vi "Main UI.vi"(11 "FormulaLV App in":refnum<class "FormulaG App.lvclass">) -> ()   [LabVIEW 2020, in "FormulaG.lvlib" / "FormulaG App.lvclass"]
uses:
  FormulaG App.lvclass
  FormulaG-Common/Camera.ctl
  <vilib>/sklein/WebView2/Webview2 Control/WebView2 Control.xctl
  FormulaG App.lvclass/FormulaG App.ctl
  FormulaG-Common/UI Options.ctl
  <vilib>/Platform/browser.llb/Open URL in Default Browser (string).vi
  HTTP Logs UI.vi
  FormulaG-Common/FormulaG-Common.lvlib
  FormulaG API/FormulaG API.lvclass
  <vilib>/IlluminatedG/IG GodotServer/GodotLV/GodotServer/GodotServer.lvclass
panel:
  out "Web":string(xcontrol)
  in  "HTTP Logs":bool
  out "Throttle":sgl(slide) scale=0.0..1.0
  out "Speed":dbl(knob) scale=0.0..10.0
  in  "Clear Map":bool
  out "Last Lap":dbl format="%<%M:%S%3u>t"
  out "Current Lap":dbl format="%<%M:%S%3u>t"
  out "XY Graph":cluster{dbl[], dbl[]}[](graph)
  in  "Pause":bool
  out "Chart":sgl[][](graph)
  in  "Camera":T1
  in  "Reset":bool
  out "Steering":sgl(knob) scale=-1.0..1.0
  out "Connected":bool
  in  "Show Range Lines":bool
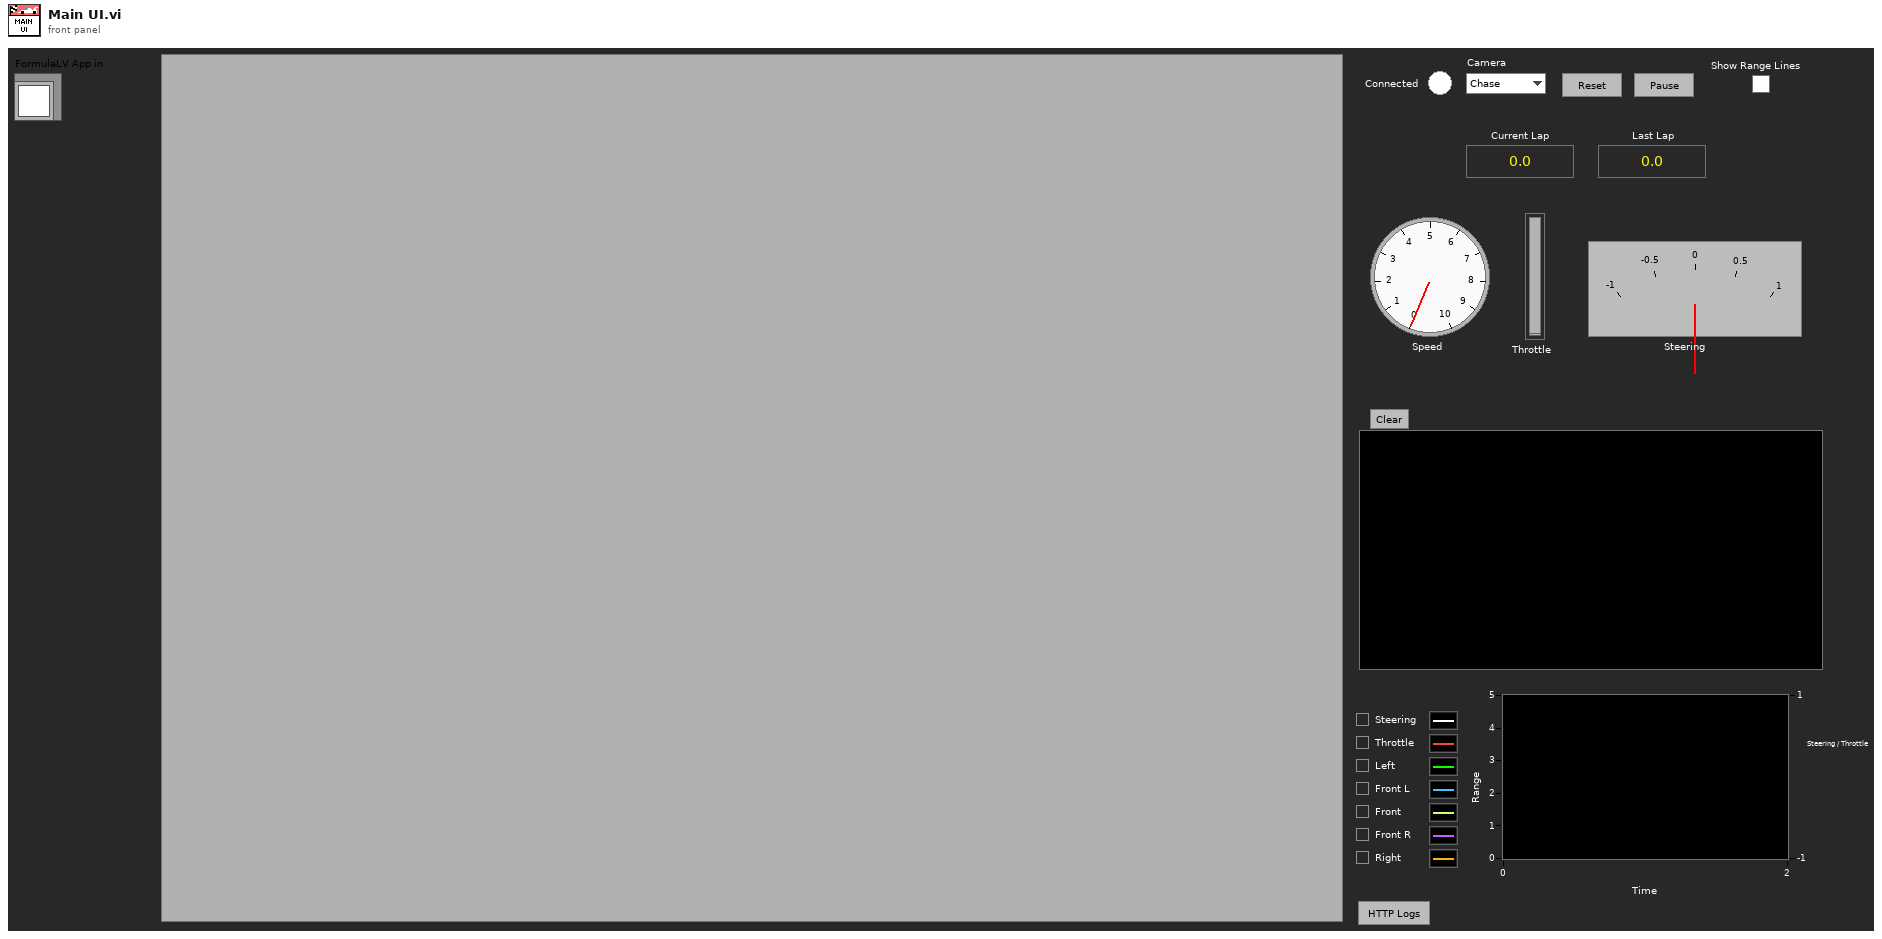
[diagram p1: front panel]
types:
  T1 = typedef "FormulaG-Common.lvlib/Camera.ctl" = enum16{"Chase", "Overhead"}
  T2 = typedef "FormulaG-Common.lvlib/UI Options.ctl" = cluster{"Range Visible":bool}
  T3 = typedef "FormulaG-Common.lvlib/Control VI.ctl" = refnum<vi>
  T4 = typedef "FormulaG-Common.lvlib/Ranges.ctl" = cluster{"Front":sgl[], "Rear":sgl[]}
  T5 = typedef "FormulaG-Common.lvlib/Car Info.ctl" = cluster{"Speed":sgl, "X":sgl, "Y":sgl, "Heading":sgl}
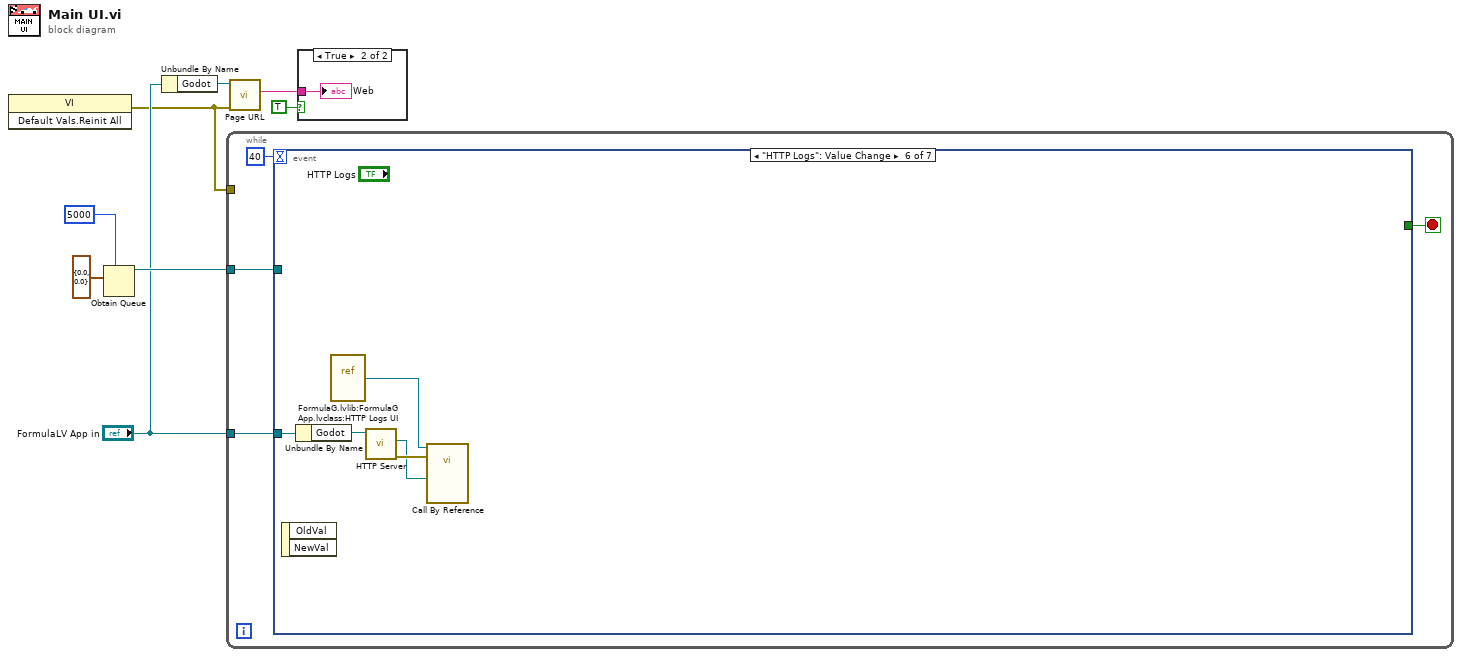
[diagram p0: block diagram]
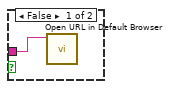
[diagram p2: hidden frame]
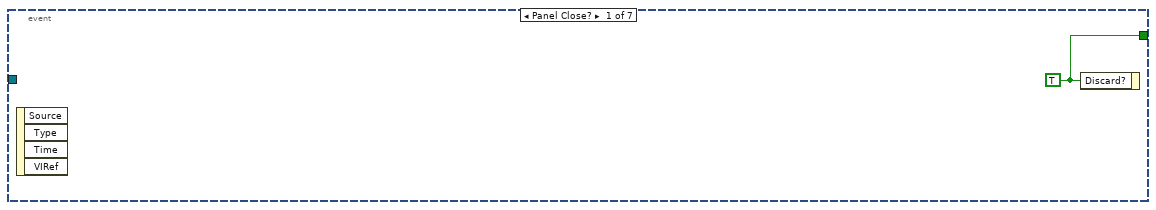
[diagram p3: hidden frame]
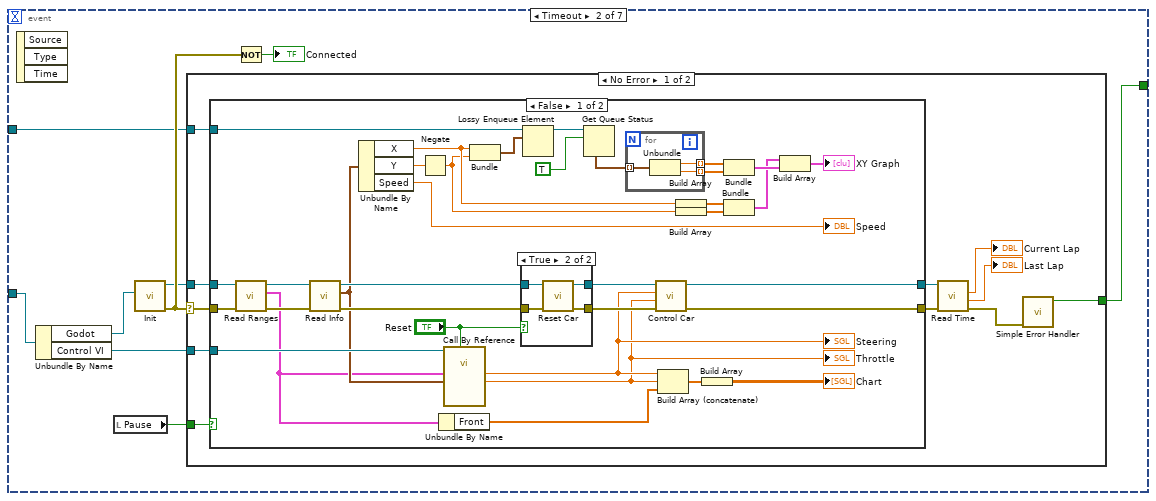
[diagram p4: hidden frame]
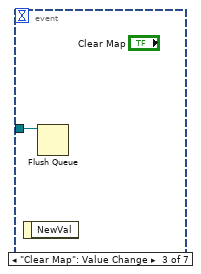
[diagram p8: hidden frame]
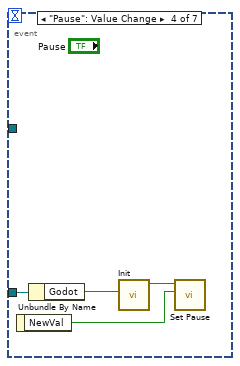
[diagram p9: hidden frame]
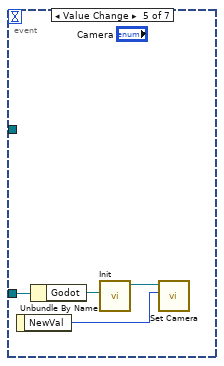
[diagram p10: hidden frame]
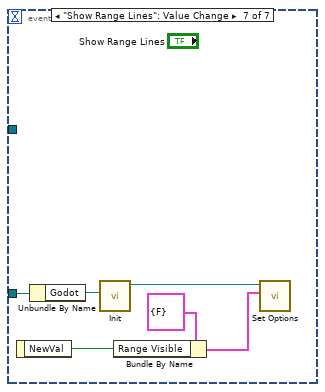
[diagram p11: hidden frame]
diagram:
  n1 = invoke class="VI" method="Default Vals.Reinit All"() -> (error out=w1:errorcluster)  [unwired: 3 in, 2 out]
  n2 = Obtain Queue(max queue size (-1, unlimited)=5000, element data type=cluster{dbl, dbl} {0.0, 0.0}) -> (queue out=w6:refnum<queue>)  [unwired: 3 in, 2 out]
  n3 = Unbundle By Name("FormulaLV App in") -> ("Godot"=w3:refnum<class "GodotServer.lvclass">)
  n4 = while {
    tunnel: "FormulaLV App in" -> [w11]
    tunnel: w1 -> [_]
    tunnel: w6 -> [w9]
    stop <- w12 stop-if-true
    n5 = event shown="[5] \"HTTP Logs\": Value Change" {
      selector: _ -> [_ _ _ _ _ _ _]
      dyn-events: _ -> [_ _ _ _ _ _ _]
      timeout: 40 -> [_ _ _ _ _ _ _]
      tunnel: [w13 w16 _ _ _ _ _] -> w12
      tunnel: w11 -> [_ w18 _ w83 w87 w92 w98]
      tunnel: w9 -> [_ w19 w79 _ _ _ _]
      event Panel Close? {
        w13 = TRUE ("Discard?")
        n6 = event-data() -> ()  [unwired: 1 in, 4 out]
        n7 = event-data("Discard?"=w13) -> ()  [unwired: 1 in, 1 out]
      }
      event Timeout {
        n8 = event-data() -> ()  [unwired: 1 in, 3 out]
        n9 = Unbundle By Name(w18) -> ("Godot"=w14:refnum<class "GodotServer.lvclass">, "Control VI"=w17:T3)
        n10 = local read "Pause"() -> (w15:bool)
        n11 = call "Init.vi"("Godot"=w14) -> ("error out"=w21:errorcluster, "FormulaG API out"=w20:refnum<class "FormulaG API.lvclass">)  [unwired: 9 in]
        n12 = case shown="No Error" w21 {
          selector: w21 -> [w30 _]
          tunnel: w20 -> [w33 _]
          tunnel: w19 -> [w32 _]
          tunnel: w17 -> [w31 _]
          tunnel: [w28 _] -> w16
          tunnel: w15 -> [w29 _]
          frame No Error {
            n13 = case shown="False" w29 {
              tunnel: w33 -> [w65 w78]
              tunnel: w32 -> [w61 _]
              tunnel: w31 -> [w47 _]
              tunnel: w30 -> [w39 _]
              tunnel: [w35 w78] -> w27
              tunnel: [w34 _] -> w26
              frame False {
                n14 = call "Read Ranges.vi"("error in (no error)"=w39, "FormulaG API in"=w65) -> ("error out"=w66:errorcluster, "Ranges"=w45:T4, "FormulaG API out"=w64:refnum<class "FormulaG API.lvclass">)  [unwired: 7 in]
                n15 = call "Read Info.vi"("error in (no error)"=w66, "FormulaG API in"=w64) -> ("error out"=w68:errorcluster, "Info"=w46:T5, "FormulaG API out"=w63:refnum<class "FormulaG API.lvclass">)  [unwired: 7 in]
                n16 = Unbundle By Name(w46) -> ("X"=w57:sgl, "Y"=w62:sgl, "Speed"=→"Speed":sgl)
                n17 = Negate(x=w62) -> (-x=w56:sgl)
                n18 = Unbundle By Name(w45) -> ("Front"=w44:sgl[])
                n19 = call-by-ref "?"(reference=w47, "Reset"="Reset", "Car Info"=w46, "Ranges"=w45) -> ("Throttle (0 to 1)"=w37:sgl, "Steering (-1 to 1)"=w41:sgl)  [unwired: 8 in, 2 out]
                "Steering" <- w41
                "Throttle" <- w37
                n20 = Bundle("X"=w57, w56) -> (w60:cluster{"X":sgl, sgl})  [unwired: 1 in]
                n21 = case shown="True" "Reset" {
                  tunnel: w63 -> [w70 w74]
                  tunnel: [w70 w73] -> w40
                  tunnel: w68 -> [w69 w72]
                  tunnel: [w69 w71] -> w67
                  frame False {
                  }
                  frame True {
                    n22 = call "Reset Car.vi"("error in (no error)"=w72, "FormulaG API in"=w74) -> ("error out"=w71:errorcluster, "FormulaG API out"=w73:refnum<class "FormulaG API.lvclass">)  [unwired: 8 in]
                  }
                }
                n23 = Lossy Enqueue Element(queue=w61, element=w60) -> (queue out=w59:refnum<queue>)  [unwired: 1 in, 3 out]
                n24 = Get Queue Status(queue=w59, return elements? (F)=TRUE) -> (elements=w55:cluster{dbl, dbl}[])  [unwired: 1 in, 7 out]
                n25 = for {
                  tunnel: w55 -> [w77] mode=indexing
                  tunnel: [w76] -> w52 mode=indexing
                  tunnel: [w75] -> w51 mode=indexing
                  n26 = Unbundle(w77) -> (w76:dbl, w75:dbl)
                }
                n27 = call "Control Car.vi"("error in (no error)"=w67, "Throttle"=w37, "Steering"=w41, "FormulaG API in"=w40) -> ("error out"=w34:errorcluster, "FormulaG API out"=w35:refnum<class "FormulaG API.lvclass">)  [unwired: 6 in]
                n28 = Build Array (concatenate)(w41, w37, w44) -> (w43:sgl[])
                n29 = Build Array(w57) -> (w54:sgl[])
                n30 = Build Array(w56) -> (w53:sgl[])
                n31 = Build Array(w43) -> (→"Chart":sgl[][])
                n32 = Bundle(w52, w51) -> (w50:cluster{dbl[], dbl[]})  [unwired: 1 in]
                n33 = Bundle(w54, w53) -> (w49:cluster{sgl[], sgl[]})  [unwired: 1 in]
                n34 = Build Array(w49, w50) -> (→"XY Graph":cluster{dbl[], dbl[]}[])
              }
              frame True {
              }
            }
            n35 = call "Read Time.vi"("error in (no error)"=w26, "FormulaG API in"=w27) -> ("error out"=w25:errorcluster, "Last Lap"=→"Last Lap":dbl, "Current Lap"=→"Current Lap":dbl)  [unwired: 6 in, 1 out]
            n36 = call <vilib>:"Simple Error Handler.vi"("error in (no error)"=w25) -> ("error?"=w28:bool)  [unwired: 4 in, 4 out]
          }
          frame Error {
          }
        }
        n37 = Not(x=w21) -> (.not. x?=→"Connected":bool)
      }
      event "Clear Map": Value Change {
        n38 = event-data() -> ()  [unwired: 1 in, 1 out]
        n39 = Flush Queue(queue=w79) -> ()  [unwired: 1 in, 3 out]
      }
      event "Pause": Value Change {
        n40 = event-data() -> ("NewVal"=w81:bool)  [unwired: 1 in]
        n41 = Unbundle By Name(w83) -> ("Godot"=w80:refnum<class "GodotServer.lvclass">)
        n42 = call "Init.vi"("Godot"=w80) -> ("FormulaG API out"=w82:refnum<class "FormulaG API.lvclass">)  [unwired: 9 in, 1 out]
        n43 = call "Set Pause.vi"("Pause"=w81, "FormulaG API in"=w82) -> ()  [unwired: 8 in, 2 out]
      }
      event Value Change {
        n44 = event-data() -> ("NewVal"=w85:T1)  [unwired: 1 in]
        n45 = Unbundle By Name(w87) -> ("Godot"=w84:refnum<class "GodotServer.lvclass">)
        n46 = call "Init.vi"("Godot"=w84) -> ("FormulaG API out"=w86:refnum<class "FormulaG API.lvclass">)  [unwired: 9 in, 1 out]
        n47 = call "Set Camera.vi"("Camera"=w85, "FormulaG API in"=w86) -> ()  [unwired: 8 in, 2 out]
      }
      event "HTTP Logs": Value Change {
        n48 = event-data() -> ()  [unwired: 1 in, 2 out]
        n49 = Unbundle By Name(w92) -> ("Godot"=w91:refnum<class "GodotServer.lvclass">)
        n50 = vi-ref "FormulaG.lvlib:FormulaG App.lvclass:HTTP Logs UI.vi"() -> (w89:refnum<vi>)
        n51 = call <vilib>:"HTTP Server.vi"("GodotServer in"=w91) -> ("error out"=w90:errorcluster, "HTTP Server"=w88:refnum<class "Server.lvclass">)  [unwired: 8 in, 1 out]
        n52 = call-by-ref "?"(reference=w89, error in=w90, "HTTP Server"=w88) -> ()  [unwired: 11 in, 2 out]
      }
      event "Show Range Lines": Value Change {
        n53 = event-data() -> ("NewVal"=w96:bool)  [unwired: 1 in]
        n54 = Unbundle By Name(w98) -> ("Godot"=w93:refnum<class "GodotServer.lvclass">)
        n55 = call "Init.vi"("Godot"=w93) -> ("FormulaG API out"=w94:refnum<class "FormulaG API.lvclass">)  [unwired: 9 in, 1 out]
        n56 = Bundle By Name(cluster=T2 {"Range Visible"=FALSE} ("UI Options"), "Range Visible"=w96) -> (w95:T2)
        n57 = call "Set Options.vi"("UI Options"=w95, "FormulaG API in"=w94) -> ()  [unwired: 8 in, 2 out]
      }
    }
  }
  n58 = call <vilib>:"Page URL.vi"("error in (no error)"=w1, "GodotServer in"=w3) -> ("Page URL"=w2:string)  [unwired: 7 in, 2 out]
  n59 = case shown="True" TRUE {
    tunnel: w2 -> [w99 w100]
    frame False {
      n60 = call-poly <vilib>:"Open URL in Default Browser.vi"("URL"=w99) -> ()  [unwired: 5 in, 2 out]
    }
    frame True {
      "Web" <- w100
    }
  }
